vi "AB Error Dialog.vi"(10 "Auto Balance State":T1) -> ()   [LabVIEW 2009]
uses:
  Autobalance Status Data.ctl
  Apps/Yes No Button.ctl
  Autobalance Stage.ctl
  Autobalance Data Point.ctl
panel:
  in  "Boolean":bool
  # "Hi - Lo Commands have\ncrossed over."
  # "Cmd"
  # "Servo"
  # "Cmd"
  # "Servo"
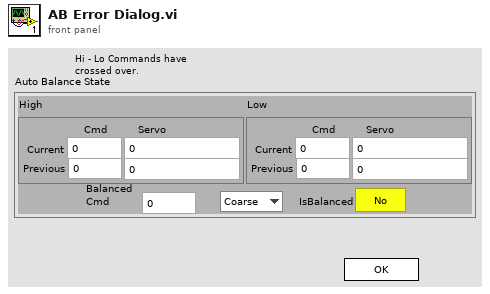
[diagram p1: front panel]
types:
  T1 = typedef "Autobalance Status Data.ctl" = cluster{"IsBalanced":T2, "Autobalance Stage":T3, "High":T4, "Low":T4, "Balanced \nCmd":dbl}
  T2 = typedef "Yes No Button.ctl" = bool
  T3 = typedef "Autobalance Stage.ctl" = enum16{"Coarse", "Fine", "Backing Up", "Done"}
  T4 = typedef "Autobalance Data Point.ctl" = cluster{"cCmd":dbl, "cServo":dbl, "pCmd":dbl, "pServo":dbl}
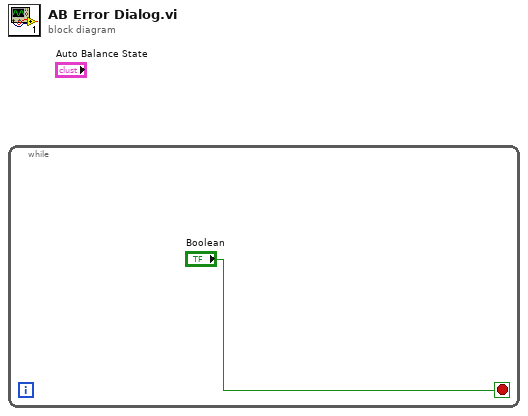
[diagram p0: block diagram]
diagram:
  n1 = while {
    stop <- "Boolean" stop-if-true
  }
